vi "Initialize.vi"(4 "Label Match Black List":string[](array[string]), 5 "Reset to Defaults":bool, 6 "Label Match White List":string[](array[string]), 7 "Tab Label in Tag":bool, 8 "error in (no error)":errorcluster, 9 "Tag Root":string, 10 "VI Refnum":refnum<vi>, 11 "UI-Bus in":refnum<class "UI-Bus.lvclass">) -> (0 "error out":errorcluster, 3 "UI-Bus out":refnum<class "UI-Bus.lvclass">)   [LabVIEW 2021, in "UI-Bus.lvclass"]
uses:
  UI-Bus.lvclass
  C:/Program Files (x86)/National Instruments/LabVIEW 2021/vi.lib/TSA/Omni-Bus/Omni-Bus/Bus Access/Bus_Access.lvclass
  UI-Bus.lvclass/UI-Bus.ctl
  <vilib>/TSA/Omni-Bus/Omni-Bus/Bus Access/Bus_Access.lvclass/Bus_Access.ctl
  <vilib>/TSA/Omni-Bus/Omni-Bus/Bus Access/Properties/Write Tag Root.vi
panel:
  # "The Black and while Lists use the Match Pattern Function to match a label.\nSo use the Match Pattern expressions to define the match\nhttps://www.ni.com/docs/en-US/bundle/labview-api-ref/page/functions/match-pattern.html\nIf both the white and black list matches then the while over rides the black list"
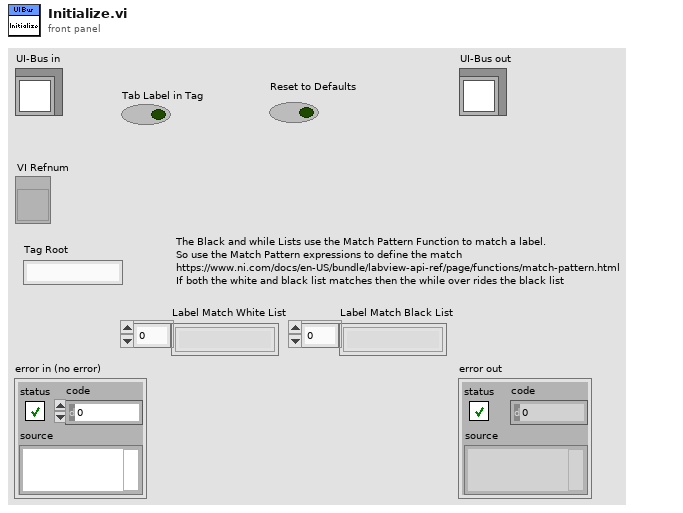
[diagram p1: front panel]
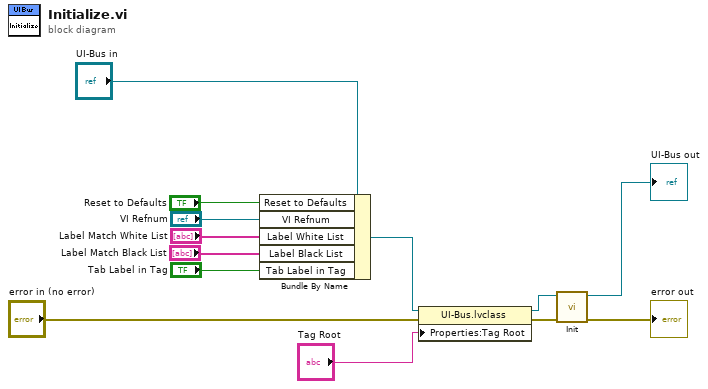
[diagram p0: block diagram]
diagram:
  n1 = Bundle By Name(cluster="UI-Bus in", "Reset to Defaults"="Reset to Defaults", "VI Refnum"="VI Refnum", "Label White List"="Label Match White List", "Label Black List"="Label Match Black List", "Tab Label in Tag"="Tab Label in Tag") -> (w4:refnum<class "UI-Bus.lvclass">)
  n2 = property class="UI-Bus.lvclass"(reference=w4, error in="error in (no error)", "Properties:Tag Root"="Tag Root") -> (reference out=w3:refnum<class "UI-Bus.lvclass">, error out=w5:errorcluster)
  n3 = call-dynamic "Init.vi"("error in (no error)"=w5, "Data in"=w3) -> ("error out"=→"error out":errorcluster, "Data out"=→"UI-Bus out":refnum<class "UI-Bus.lvclass">)  [unwired: 8 in]
